vi "Dequeue Message.vi"(8 "Error In":errorcluster, 11 "Message Queue In":refnum<queue>) -> (0 "Error Out":errorcluster, 1 "Data":variant, 2 "Command":string, 3 "Message Queue Out":refnum<queue>)   [LabVIEW 2017, in "Graveyard.lvlib"]
uses:
  Graveyard.lvlib
  Message.ctl
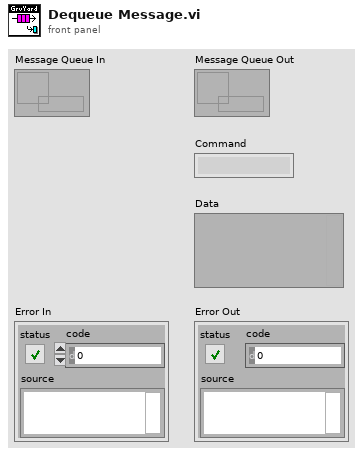
[diagram p1: front panel]
types:
  T1 = typedef "Graveyard.lvlib/Message.ctl" = cluster{"Command":string, "Data":variant}
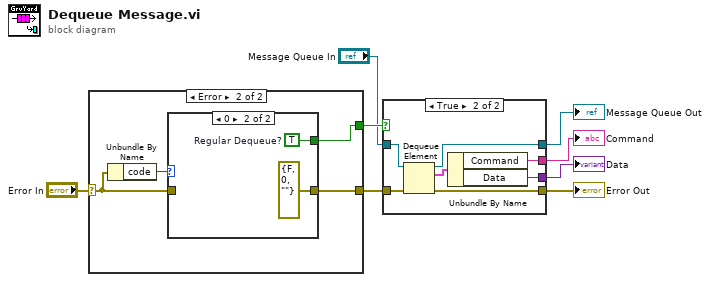
[diagram p0: block diagram]
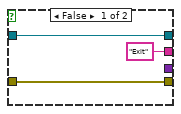
[diagram p2: hidden frame]
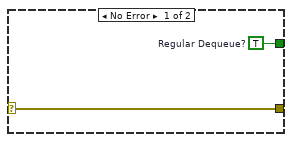
[diagram p3: hidden frame]
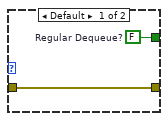
[diagram p4: hidden frame]
diagram:
  n1 = case shown="Error" "Error In" {
    selector: "Error In" -> [w10 w11]
    tunnel: [w10 w12] -> w7
    tunnel: [w9 w13] -> w6
    frame No Error {
      w9 = TRUE  # Regular Dequeue?
    }
    frame Error {
      n2 = Unbundle By Name(w11) -> ("code"=w14:i32)
      n3 = case shown="0" w14 {
        tunnel: [w16 w18] -> w13
        tunnel: [w15 errorcluster {"status"=FALSE, "code"=0, "source"=""} ("error constant")] -> w12
        tunnel: w11 -> [w15 _]
        frame Default {
          w16 = FALSE  # Regular Dequeue?
        }
        frame 0 {
          w18 = TRUE  # Regular Dequeue?
        }
      }
    }
  }
  n4 = case shown="True" w6 {
    tunnel: w7 -> [w19 w28]
    tunnel: "Message Queue In" -> [w20 w27]
    tunnel: [w20 w26] -> w4
    tunnel: ["Exit" ("Command") w24] -> w3
    tunnel: [_ w23] -> w2
    tunnel: [w19 w22] -> w1
    frame False {
    }
    frame True {
      n5 = Dequeue Element(queue=w27, error in (no error)=w28) -> (queue out=w26:refnum<queue>, element=w25:T1, error out=w22:errorcluster)  [unwired: 1 in, 1 out]
      n6 = Unbundle By Name(w25) -> ("Command"=w24:string, "Data"=w23:variant)
    }
  }
  "Message Queue Out" <- w4
  "Command" <- w3
  "Data" <- w2
  "Error Out" <- w1
